vi "set_position.vi"(8 "error in (no error)":errorcluster, 10 "last position":dbl, 11 "_delayStageBase in":refnum<class "_delayStageBase.lvclass">) -> (0 "error out":errorcluster, 3 "_delayStageBase out":refnum<class "_delayStageBase.lvclass">)   [LabVIEW 2018, in "_delayStageBase.lvclass"]
uses:
  _delayStageBase.lvclass
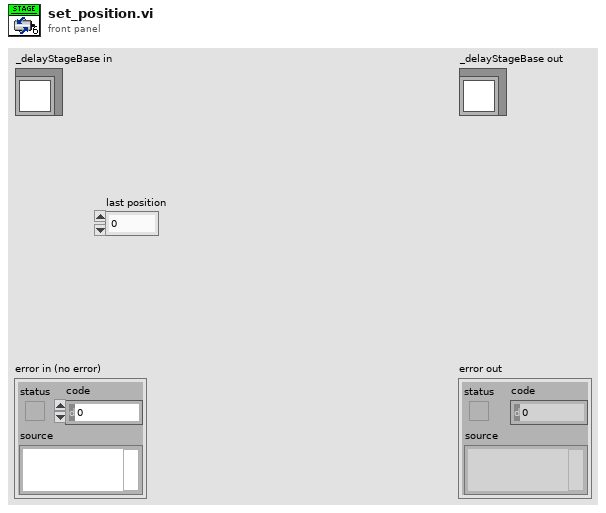
[diagram p1: front panel]
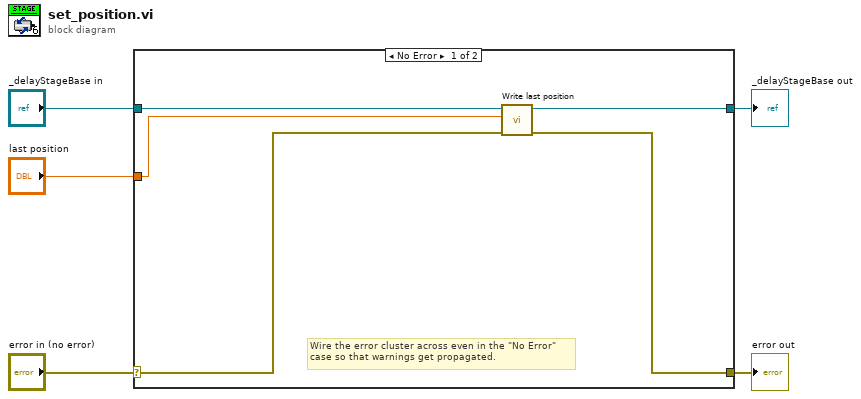
[diagram p0: block diagram]
diagram:
  n1 = case shown="No Error" "error in (no error)" {
    selector: "error in (no error)" -> [w7 w12]
    tunnel: [w6 w12] -> w4
    tunnel: [w9 w11] -> w2
    tunnel: "_delayStageBase in" -> [w10 w11]
    tunnel: "last position" -> [w8 _]
    frame No Error {
      # "Wire the error cluster across even in the \"No Error\"\ncase so that warnings get propagated."
      n2 = call-dynamic "Write last position.vi"("error in (no error)"=w7, "last position"=w8, "_delayStageBase in"=w10) -> ("error out"=w6:errorcluster, "_delayStageBase out"=w9:refnum<class "_delayStageBase.lvclass">)  [unwired: 7 in]
    }
    frame Error {
    }
  }
  "error out" <- w4
  "_delayStageBase out" <- w2
